vi "xxxx Core.vi"(8 "error in (no error)":errorcluster, 11 "Context State in":refnum<class "Context State.lvclass">) -> (0 "error out":errorcluster, 3 "Context State out":refnum<class "Context State.lvclass">)   [LabVIEW 2021, in "Context.lvlib" / "Context State.lvclass"]
uses:
  Context State.lvclass
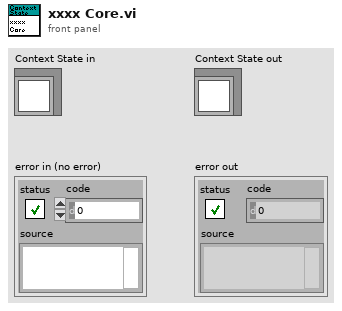
[diagram p1: front panel]
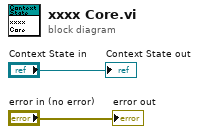
[diagram p0: block diagram]
diagram:
  "error out" <- "error in (no error)"
  "Context State out" <- "Context State in"
